vi "PulseGenEPTx_5Inj.vi"(0 "EPTxSupervisor":T2, 1 "Inj_Config_Channel3":T1, 2 "Inj_Config_Channel2":T1, 3 "Inj_Config_Channel1":T1) -> (7 "CmdOut3":bool, 8 "CmdOut2":bool, 9 "CmdOut1":bool)   [LabVIEW 2015, in "ECS-FPGA.lvlib"]
doc: "This VI is used to generate a sequence of up to five angle-based injection pulses for each channel of the DI Driver module. Each Inj_Config cluster is configured for an overall window of operation, individual pulse enabling, injection pulse start-angle, and pulse duration. This VI is supervised by the EPTxSupervisor cluster. When this VI is used in conjunction with the NI Powertrain Controls 9751 DI Driver module, the operating windows for each channel must not overlap due to DI channel multiplexing."
uses:
  ECS-FPGA.lvlib
  <vilib>/Powertrain Controls/Device Drivers/Engine Position Tracking/EPTx/RevA/FPGA/Controls/EPTxSupervisor.ctl
  <vilib>/Powertrain Controls/Device Drivers/Engine Position Tracking/EPTx/RevA/FPGA/Controls/EPTxAAPControl.ctl
  <vilib>/Powertrain Controls/Device Drivers/Engine Position Tracking/EPTx/RevA/FPGA/Extras/Command Sequence - 16e.vi
  <vilib>/Powertrain Controls/Device Drivers/Engine Position Tracking/EPTx/RevA/FPGA/Extras/Angle One Shot - 8x - Single.vi
  <vilib>/Powertrain Controls/Device Drivers/Engine Position Tracking/EPTx/RevA/FPGA/EPTx - RevA - FPGA.lvlib
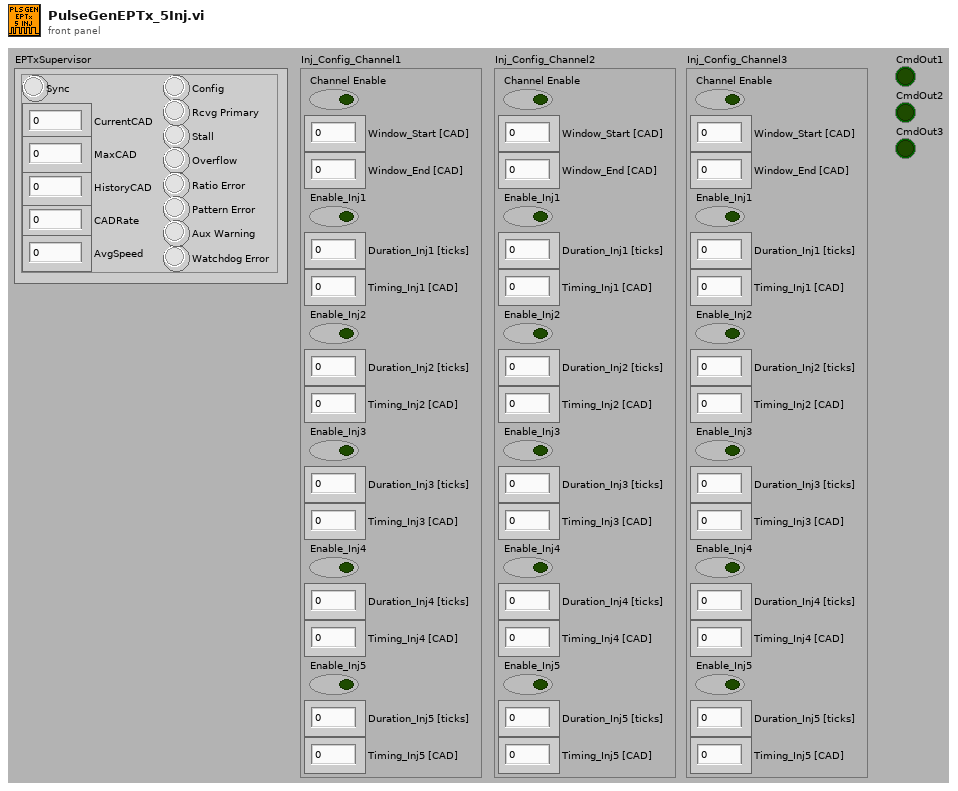
[diagram p1: front panel]
types:
  T1 = cluster{"Channel Enable":bool, "Window_Start [CAD]":fxp<+,18,11>, "Window_End [CAD]":fxp<+,18,11>, "Enable_Inj1":bool, "Duration_Inj1 [ticks]":u32, "Timing_Inj1 [CAD]":fxp<+,18,11>, "Enable_Inj2":bool, "Duration_Inj2 [ticks]":u32, "Timing_Inj2 [CAD]":fxp<+,18,11>, "Enable_Inj3":bool, "Duration_Inj3 [ticks]":u32, "Timing_Inj3 [CAD]":fxp<+,18,11>, "Enable_Inj4":bool, "Duration_Inj4 [ticks]":u32, "Timing_Inj4 [CAD]":fxp<+,18,11>, "Enable_Inj5":bool, "Duration_Inj5 [ticks]":u32, "Timing_Inj5 [CAD]":fxp<+,18,11>}
  T2 = typedef "EPTx - RevA - FPGA.lvlib/EPTxSupervisor.ctl" = cluster{"Sync":bool, "CurrentCAD":fxp<+,18,11>, "MaxCAD":fxp<+,11,11>, "HistoryCAD":fxp<+,11,11>, "CADRate":fxp<+,22,8>, "AvgSpeed":fxp<+,17,15>, "Config":bool, "Rcvg Primary":bool, "Stall":bool, "Overflow":bool, "Ratio Error":bool, "Pattern Error":bool, "Aux Warning":bool, "Watchdog Error":bool}
  T3 = typedef "EPTx - RevA - FPGA.lvlib/EPTxAAPControl.ctl" = cluster{"Enable":bool, "RisingCAD":fxp<+,18,11>, "FallingCAD":fxp<+,18,11>}
  T4 = typedef "EPTx - RevA - FPGA.lvlib/EPTxAOSControl.ctl" = cluster{"Enable":bool, "OneShotCAD":fxp<+,18,11>}
  T5 = cluster{"DurationSeq":u32[], "CmdLevelSeq":bool[], "ContinueSeq":bool[]}
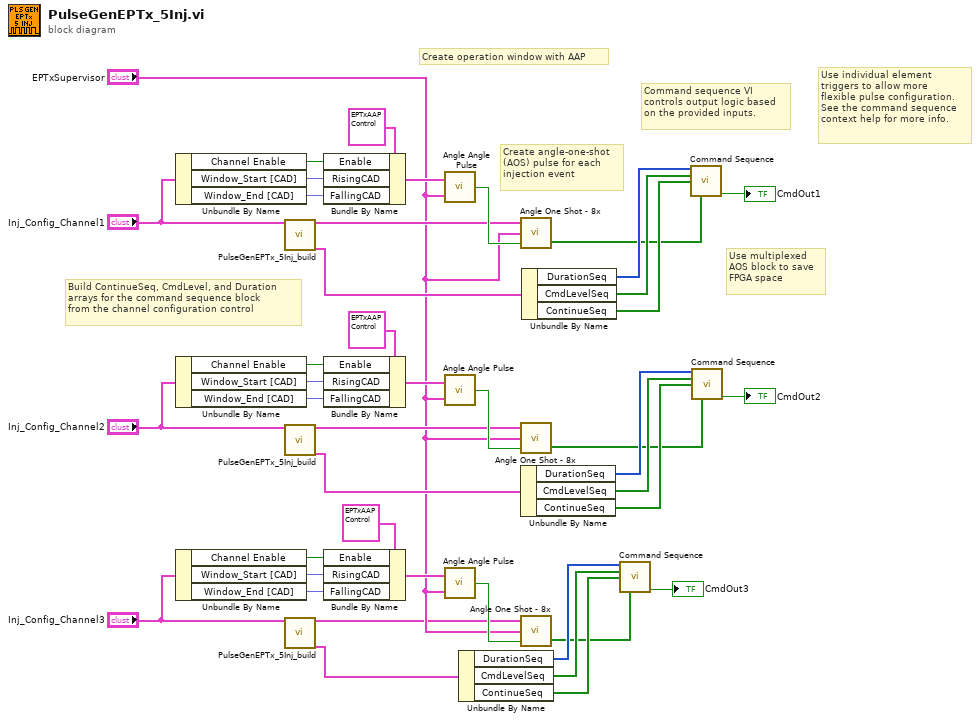
[diagram p0: block diagram]
diagram:
  # "Use individual element \ntriggers to allow more\nflexible pulse configuration.\nSee the command sequence\ncontext help for more info."
  # "Use multiplexed\nAOS block to save\nFPGA space"
  # "Command sequence VI\ncontrols output logic based\non the provided inputs."
  # "Create angle-one-shot\n(AOS) pulse for each \ninjection event"
  # "Build ContinueSeq, CmdLevel, and Duration\narrays for the command sequence block\nfrom the channel configuration control"
  # "Create operation window with AAP"
  n1 = Unbundle By Name("Inj_Config_Channel1") -> ("Channel Enable"=w35:bool, "Window_Start [CAD]"=w43:fxp<+,18,11>, "Window_End [CAD]"=w42:fxp<+,18,11>)
  n2 = Unbundle By Name("Inj_Config_Channel2") -> ("Channel Enable"=w20:bool, "Window_Start [CAD]"=w17:fxp<+,18,11>, "Window_End [CAD]"=w18:fxp<+,18,11>)
  n3 = Unbundle By Name("Inj_Config_Channel3") -> ("Channel Enable"=w11:bool, "Window_Start [CAD]"=w14:fxp<+,18,11>, "Window_End [CAD]"=w13:fxp<+,18,11>)
  n4 = call "PulseGenEPTx_5Inj_build.vi"("PlsGenConfig"="Inj_Config_Channel1") -> ("OneShotArray"=w3:T4[], "Command Seq Output"=w41:T5)  [unwired: 17 in]
  n5 = call "PulseGenEPTx_5Inj_build.vi"("PlsGenConfig"="Inj_Config_Channel2") -> ("OneShotArray"=w4:T4[], "Command Seq Output"=w16:T5)  [unwired: 17 in]
  n6 = call "PulseGenEPTx_5Inj_build.vi"("PlsGenConfig"="Inj_Config_Channel3") -> ("OneShotArray"=w1:T4[], "Command Seq Output"=w8:T5)  [unwired: 17 in]
  n7 = Bundle By Name(cluster=T3 {"Enable"=FALSE, "RisingCAD"=0.0, "FallingCAD"=0.0} ("AAPControl"), "Enable"=w35, "RisingCAD"=w43, "FallingCAD"=w42) -> (w38:T3)
  n8 = Bundle By Name(cluster=T3 {"Enable"=FALSE, "RisingCAD"=0.0, "FallingCAD"=0.0} ("AAPControl"), "Enable"=w20, "RisingCAD"=w17, "FallingCAD"=w18) -> (w19:T3)
  n9 = Bundle By Name(cluster=T3 {"Enable"=FALSE, "RisingCAD"=0.0, "FallingCAD"=0.0} ("AAPControl"), "Enable"=w11, "RisingCAD"=w14, "FallingCAD"=w13) -> (w12:T3)
  n10 = call <vilib>:"Angle Angle Pulse.vi"("EPTxSupervisor"="EPTxSupervisor", "AAPControl"=w38) -> ("AAP"=w24:bool)
  n11 = call <vilib>:"Angle Angle Pulse.vi"("EPTxSupervisor"="EPTxSupervisor", "AAPControl"=w19) -> ("AAP"=w22:bool)
  n12 = call <vilib>:"Angle Angle Pulse.vi"("EPTxSupervisor"="EPTxSupervisor", "AAPControl"=w12) -> ("AAP"=w9:bool)
  n13 = Unbundle By Name(w8) -> ("DurationSeq"=w30:u32[], "CmdLevelSeq"=w29:bool[], "ContinueSeq"=w28:bool[])
  n14 = call-poly <vilib>:"Angle One Shot - 8x.vi"("OpWindow"=w24, "EPTxSupervisor"="EPTxSupervisor", "AOSControl"=w3) -> ("AOS"=w23:bool[])  [unwired: 1 in]
  n15 = call-poly <vilib>:"Angle One Shot - 8x.vi"("OpWindow"=w22, "EPTxSupervisor"="EPTxSupervisor", "AOSControl"=w4) -> ("AOS"=w15:bool[])  [unwired: 1 in]
  n16 = Unbundle By Name(w16) -> ("DurationSeq"=w32:u32[], "CmdLevelSeq"=w33:bool[], "ContinueSeq"=w34:bool[])
  n17 = call-poly <vilib>:"Angle One Shot - 8x.vi"("OpWindow"=w9, "EPTxSupervisor"="EPTxSupervisor", "AOSControl"=w1) -> ("AOS"=w7:bool[])  [unwired: 1 in]
  n18 = Unbundle By Name(w41) -> ("DurationSeq"=w40:u32[], "CmdLevelSeq"=w39:bool[], "ContinueSeq"=w37:bool[])
  n19 = call-poly <vilib>:"Command Sequence.vi"("DurationSeq"=w30, "CmdLevelSeq"=w29, "ContinueSeq"=w28, "ElementTriggers"=w7) -> ("Cmd"=→"CmdOut3":bool)  [unwired: 8 in, 3 out]
  n20 = call-poly <vilib>:"Command Sequence.vi"("DurationSeq"=w40, "CmdLevelSeq"=w39, "ContinueSeq"=w37, "ElementTriggers"=w23) -> ("Cmd"=→"CmdOut1":bool)  [unwired: 8 in, 3 out]
  n21 = call-poly <vilib>:"Command Sequence.vi"("DurationSeq"=w32, "CmdLevelSeq"=w33, "ContinueSeq"=w34, "ElementTriggers"=w15) -> ("Cmd"=→"CmdOut2":bool)  [unwired: 8 in, 3 out]
